vi "Set Event HMI Autotest.vi"(8 "error in (no error)":errorcluster caption="entrée d'erreur (pas d'erreur)", 10 "Event Autotest":refnum<user-event>, 11 "Actor_Autotest en entrée":refnum<class "Actor_Autotest.lvclass">) -> (0 "error out":errorcluster caption="sortie d'erreur", 3 "Actor_Autotest en sortie":refnum<class "Actor_Autotest.lvclass">)   [LabVIEW 2020, in "Library Core.lvlib" / "Actor_Autotest.lvlib" / "Actor_Autotest.lvclass"]
uses:
  Actor_Autotest.lvclass
  Instrument/Instrument (Default)/Class Instrument (Default).lvclass
  Commun VI/TypeDef/Commande Popup autotest/Commande element autotest.ctl
  Actor_Autotest.lvclass/Actor_Autotest.ctl
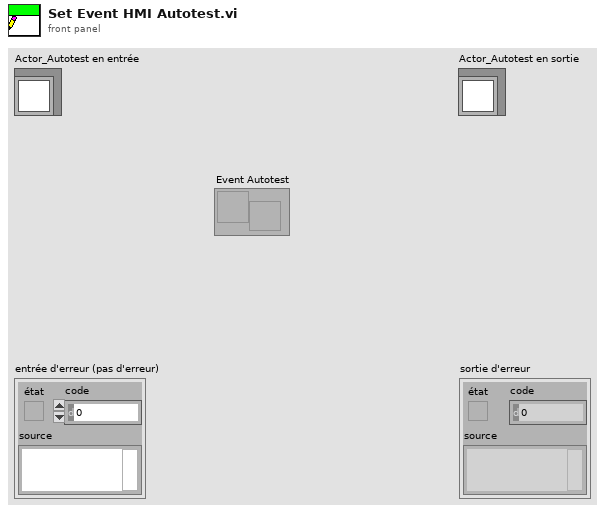
[diagram p1: front panel]
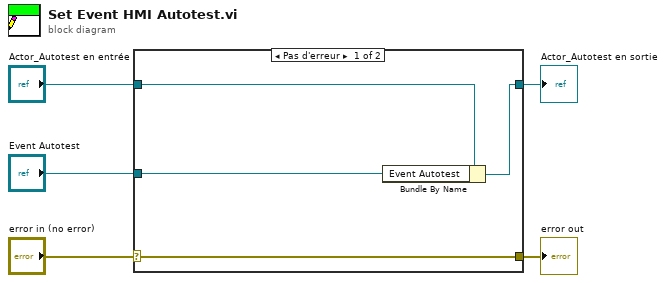
[diagram p0: block diagram]
diagram:
  n1 = case shown="Pas d'erreur" "error in (no error)" {
    selector: "error in (no error)" -> [w9 w10]
    tunnel: [w9 w10] -> w4
    tunnel: [w7 w11] -> w2
    tunnel: "Actor_Autotest en entrée" -> [w8 w11]
    tunnel: "Event Autotest" -> [w6 _]
    frame No Error {
      n2 = Bundle By Name(cluster=w8, "Event Autotest"=w6) -> (w7:refnum<class "Actor_Autotest.lvclass">)
    }
    frame Error {
    }
  }
  "error out" <- w4
  "Actor_Autotest en sortie" <- w2
